vi "vision.vi"(0 "Image 3":T1(plugin-control), 1 "Color Plane":i32) -> ()   [LabVIEW 2018]
uses:
  Vision info.vi
panel:
  out "Circles 2":cluster{"x":dbl, "y":dbl, "r":dbl}[](array[cluster])
  out "cube found":bool
  out "Type":enum16{"Z", "I", "O", "S", "L", "J", "T", "N"}(ring)=enum."O"
  out "Discriptor":dbl[](array[numeric])
  out "Image 2":T1(plugin-control)
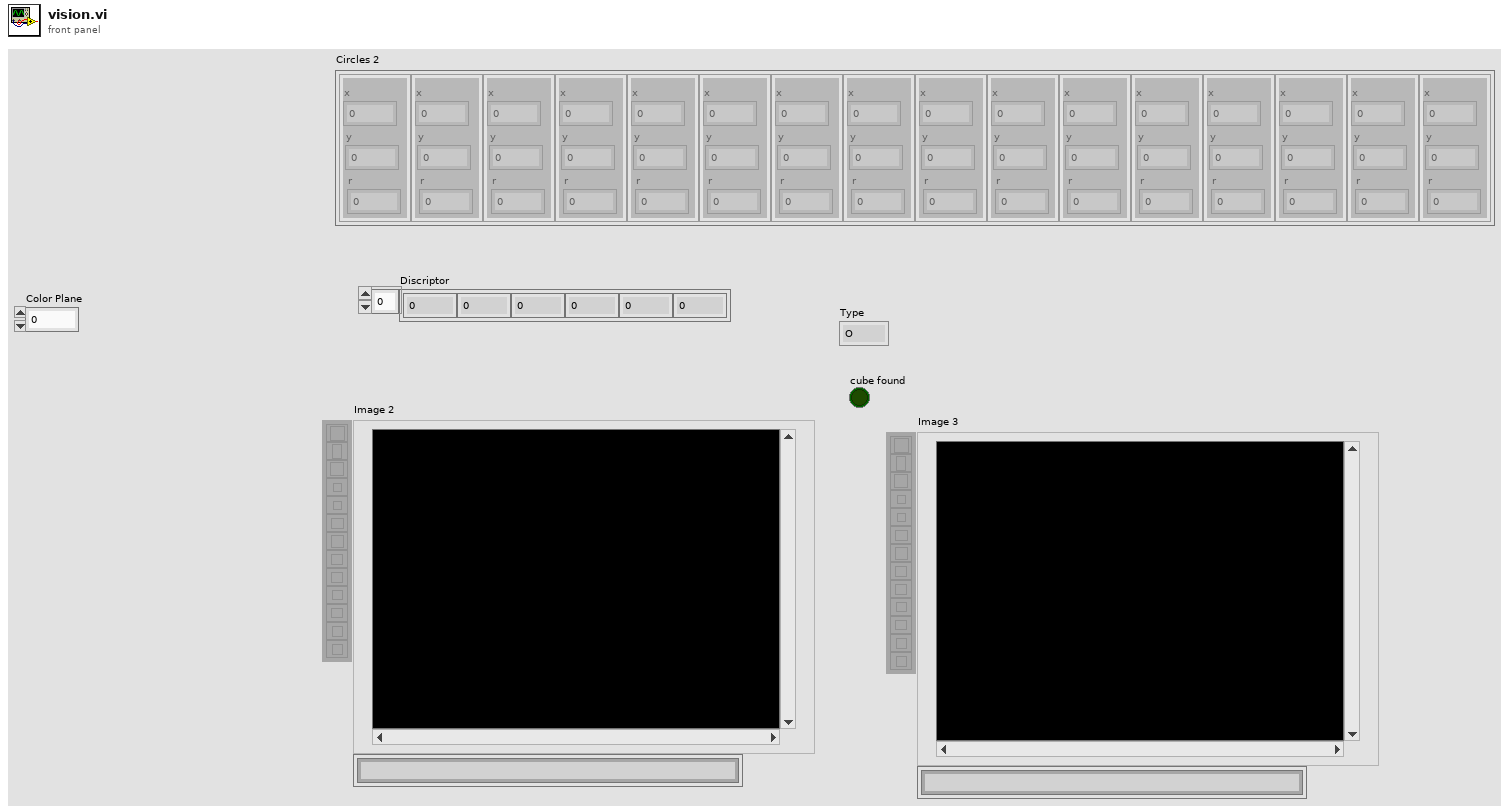
[diagram p1: front panel]
types:
  T1 = typedef "IMAQ Image.ctl" = refnum<image>
  T2 = cluster{"p1":cluster{"x":dbl, "y":dbl}, "p2":cluster{"x":dbl, "y":dbl}}
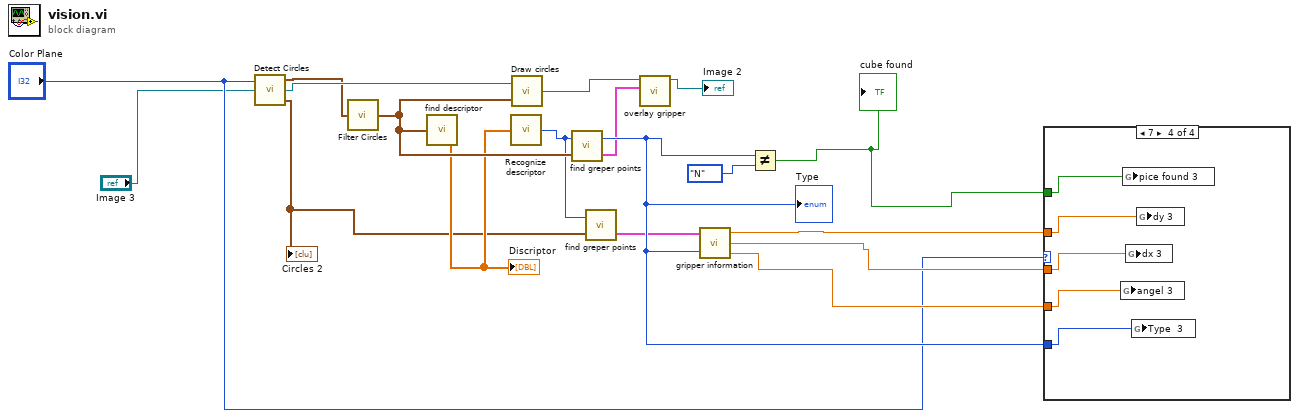
[diagram p0: block diagram]
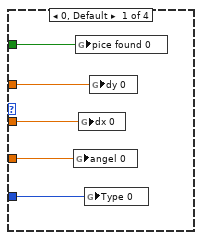
[diagram p2: hidden frame]
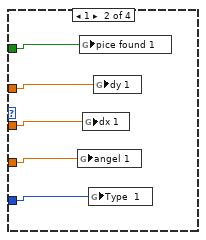
[diagram p3: hidden frame]
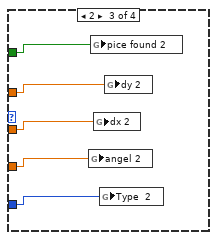
[diagram p4: hidden frame]
diagram:
  n1 = call "Detect Circles.vi"("Image 3"="Image 3", "Color Plane"="Color Plane") -> ("Circles 2"=w5:cluster{"x":dbl, "y":dbl, "r":dbl}[], "Image 4"=w3:T1, "Circles"=w2:cluster{"x":dbl, "y":dbl, "r":dbl}[])  [unwired: 1 in]
  "Circles 2" <- w5
  n2 = call "Filter Circles.vi"("Circles"=w2) -> ("out"=w12:cluster{"x":dbl, "y":dbl, "r":dbl}[])
  n3 = call "find descriptor.vi"("Circles"=w12) -> ("d"=w9:dbl[])
  "Discriptor" <- w9
  n4 = call "Recognize descriptor.vi"("Discriptor"=w9) -> ("Type"=w6:enum16{"Z", "I", "O", "S", "L", "J", "T", "N"})
  n5 = call "Draw circles .vi"("Circles"=w12, "Refnum in"=w3) -> ("Refnum out"=w8:T1)
  n6 = call "find greper points.vi"("Circles"=w12, "Type  2"=w6) -> ("gripper"=w10:T2, "Type"=w18:enum16{"Z", "I", "O", "S", "L", "J", "T", "N"})
  "Type" <- w18
  n7 = call "find greper points.vi"("Circles"=w5, "Type  2"=w6) -> ("gripper"=w4:T2)  [unwired: 1 out]
  n8 = call "overlay gripper.vi"("gripper"=w10, "Refnum in"=w8) -> ("Refnum out"=→"Image 2":T1)  [unwired: 9 in]
  n9 = call "gripper information.vi"("gripper"=w4, "Type"=w18) -> ("dy"=w15:dbl, "dx"=w16:dbl, "Angel"=w17:dbl)
  n10 = Not Equal?(x=w18, y=enum16{"Z", "I", "O", "S", "L", "J", "T", "N"}."N") -> (x != y?=w14:bool)
  "cube found" <- w14
  n11 = case shown="7" "Color Plane" {
    tunnel: w14 -> [w23 w28 w33 w38]
    tunnel: w15 -> [w22 w27 w32 w37]
    tunnel: w16 -> [w21 w26 w31 w36]
    tunnel: w17 -> [w20 w25 w30 w35]
    tunnel: w18 -> [w19 w24 w29 w34]
    frame 0, Default {
      n12 = global write "Vision info.vi" "angel 0"(w20) -> ()
      n13 = global write "Vision info.vi" "pice found 0"(w23) -> ()
      n14 = global write "Vision info.vi" "dx 0"(w21) -> ()
      n15 = global write "Vision info.vi" "Type 0"(w19) -> ()
      n16 = global write "Vision info.vi" "dy 0"(w22) -> ()
    }
    frame 1 {
      n17 = global write "Vision info.vi" "angel 1"(w25) -> ()
      n18 = global write "Vision info.vi" "pice found 1"(w28) -> ()
      n19 = global write "Vision info.vi" "dx 1"(w26) -> ()
      n20 = global write "Vision info.vi" "Type  1"(w24) -> ()
      n21 = global write "Vision info.vi" "dy 1"(w27) -> ()
    }
    frame 2 {
      n22 = global write "Vision info.vi" "angel 2"(w30) -> ()
      n23 = global write "Vision info.vi" "pice found 2"(w33) -> ()
      n24 = global write "Vision info.vi" "dx 2"(w31) -> ()
      n25 = global write "Vision info.vi" "Type  2"(w29) -> ()
      n26 = global write "Vision info.vi" "dy 2"(w32) -> ()
    }
    frame 7 {
      n27 = global write "Vision info.vi" "angel 3"(w35) -> ()
      n28 = global write "Vision info.vi" "pice found 3"(w38) -> ()
      n29 = global write "Vision info.vi" "dx 3"(w36) -> ()
      n30 = global write "Vision info.vi" "Type  3"(w34) -> ()
      n31 = global write "Vision info.vi" "dy 3"(w37) -> ()
    }
  }
